vi "Read Resistance Configuration.vi"(8 "error in (no error)":errorcluster, 11 "BNT_DMQmx-MCSV-RTD in":refnum<class "BNT_DMQmx-MCSV-RTD.lvclass">) -> (0 "error out":errorcluster, 2 "Resistance Configuration":i32(ring)=2 items=["2-Wire"=2, "3-Wire"=3, "4-Wire"=4], 3 "BNT_DMQmx-MCSV-RTD out":refnum<class "BNT_DMQmx-MCSV-RTD.lvclass">)   [LabVIEW 2016, in "BNT_DAQmx.lvlib" / "BNT_DMQmx-MCSV-RTD.lvclass"]
doc: "Read Resistance Configuration."
uses:
  BNT_DMQmx-MCSV-RTD.lvclass
  BNT_DMQmx-MCSV-RTD.lvclass/BNT_DMQmx-MCSV-RTD.ctl
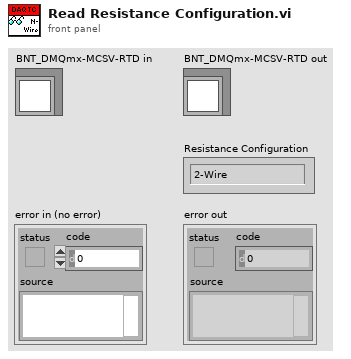
[diagram p1: front panel]
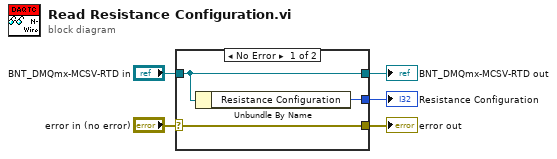
[diagram p0: block diagram]
diagram:
  n1 = case shown="No Error" "error in (no error)" {
    selector: "error in (no error)" -> [w8 w9]
    tunnel: [w8 w9] -> w4
    tunnel: [w7 w10] -> w2
    tunnel: "BNT_DMQmx-MCSV-RTD in" -> [w7 w10]
    tunnel: [w6 _] -> w1
    frame No Error {
      n2 = Unbundle By Name(w7) -> ("Resistance Configuration"=w6:i32)
    }
    frame Error {
    }
  }
  "error out" <- w4
  "BNT_DMQmx-MCSV-RTD out" <- w2
  "Resistance Configuration" <- w1
